vi "test_moteur.vi"() -> ()   [LabVIEW 2023]
panel:
  in  "WRITE PARAM":bool
  in  "param":T1
  out "param out":T1
  in  "READ PARAM":bool
  out "error out 2":errorcluster
  out "Serial Settings:Number of Bytes at Serial Port":u32
  in  "READ":bool
  out "read buffer":string
  in  "WRITE":bool
  in  "stop":bool
  in  "write buffer":string
  in  "VISA resource name":refnum<visa-resource-name>
  out "error out":errorcluster
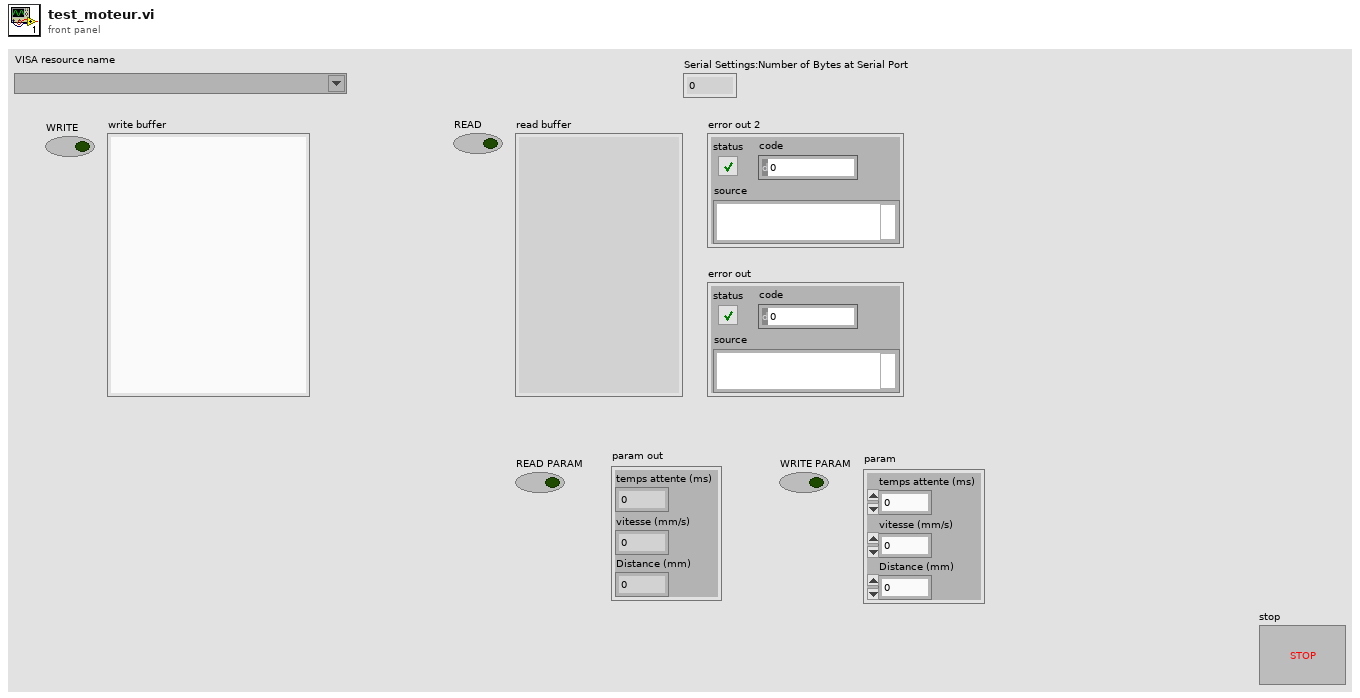
[diagram p1: front panel]
types:
  T1 = cluster{"temps attente (ms)":i32, "vitesse (mm/s)":dbl, "Distance (mm)":dbl}
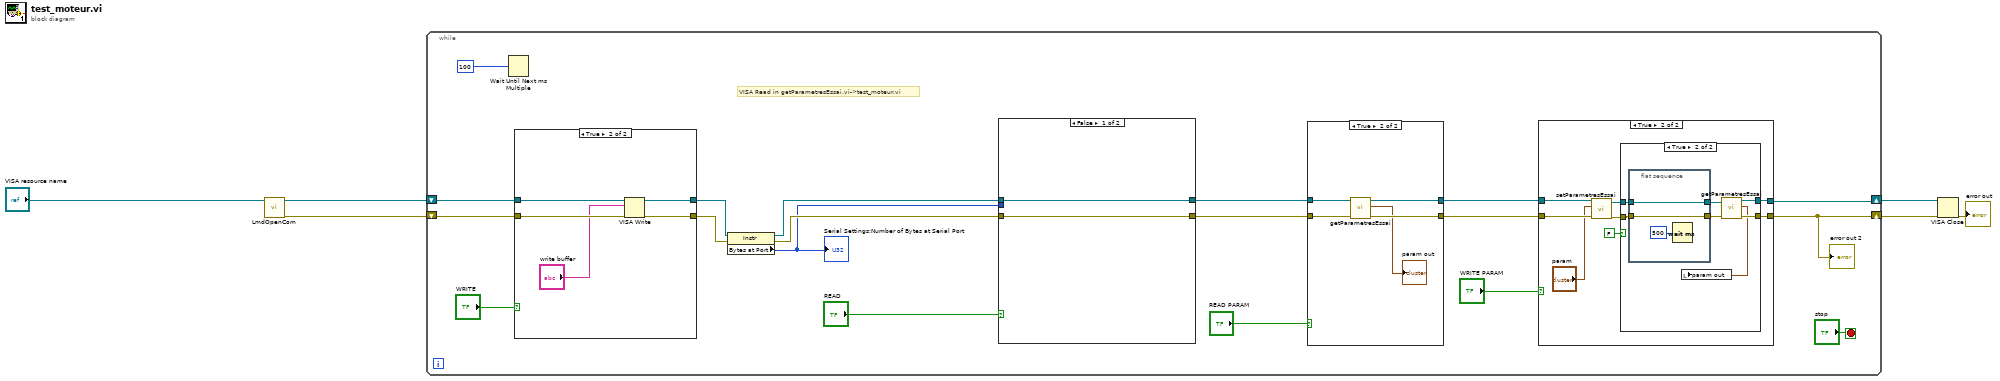
[diagram p0: block diagram]
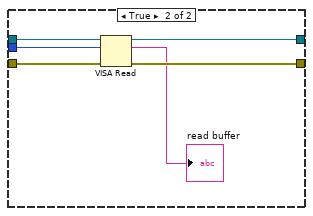
[diagram p5: hidden frame]
diagram:
  n1 = call "LmdOpenCom.vi"("VISA Refnum in"="VISA resource name") -> ("error out"=w5:errorcluster, "VISA Refnum out"=w1:refnum<visa-resource-name>)  [unwired: 9 in]
  n2 = while {
    shift-right: [w8] -> w3
    shift-left: w1 -> [w25]
    shift-right: [w9] -> w4
    shift-left: w5 -> [w24]
    stop <- "stop" stop-if-true
    # "VISA Read in getParametresEssai.vi->test_moteur.vi"
    n3 = Wait Until Next ms Multiple(millisecond multiple=u32 100) -> ()  [unwired: 1 out]
    n4 = case shown="True" "WRITE" {
      tunnel: w25 -> [w64 w69]
      tunnel: w24 -> [w63 w68]
      tunnel: [w63 w67] -> w19
      tunnel: [w64 w66] -> w20
      frame False {
      }
      frame True {
        n5 = VISA Write(VISA resource name=w69, write buffer="write buffer", error in (no error)=w68) -> (VISA resource name out=w66:refnum<visa-resource-name>, error out=w67:errorcluster)  [unwired: 1 out]
      }
    }
    n6 = property class="Instr"(reference=w20, error in=w19) -> (reference out=w17:refnum<visa-resource-name>, error out=w18:errorcluster, "Bytes at Port"=w15:u32)
    "Serial Settings:Number of Bytes at Serial Port" <- w15
    n7 = case shown="False" "READ" {
      tunnel: [w56 w60] -> w13
      tunnel: w18 -> [w56 w61]
      tunnel: [w55 w59] -> w12
      tunnel: w17 -> [w55 w62]
      tunnel: w15 -> [_ w57]
      frame False {
      }
      frame True {
        n8 = VISA Read(VISA resource name=w62, byte count=w57, error in (no error)=w61) -> (VISA resource name out=w59:refnum<visa-resource-name>, read buffer=→"read buffer":string, error out=w60:errorcluster)  [unwired: 1 out]
      }
    }
    n9 = case shown="True" "READ PARAM" {
      tunnel: w13 -> [w48 w54]
      tunnel: w12 -> [w49 w53]
      tunnel: [w49 w52] -> w10
      tunnel: [w48 w51] -> w11
      frame False {
      }
      frame True {
        n10 = call "getParametresEssai.vi"("error in (no error)"=w54, "VISA resource name"=w53) -> ("error out"=w51:errorcluster, "param out"=→"param out":T1, "VISA resource name out"=w52:refnum<visa-resource-name>)  [unwired: 7 in]
      }
    }
    n11 = case shown="True" "WRITE PARAM" {
      tunnel: w11 -> [w26 w35]
      tunnel: w10 -> [w27 w34]
      tunnel: [w26 w31] -> w9
      tunnel: [w27 w32] -> w8
      frame False {
      }
      frame True {
        n12 = call "setParametresEssai.vi"("error in (no error)"=w35, "param"="param", "VISA resource name"=w34) -> ("error out"=w29:errorcluster, "VISA resource name out"=w30:refnum<visa-resource-name>)  [unwired: 7 in]
        n13 = case shown="True" FALSE {
          tunnel: [w37 w44] -> w32
          tunnel: [w36 w43] -> w31
          tunnel: w30 -> [w37 w41]
          tunnel: w29 -> [w36 w38]
          frame False {
          }
          frame True {
            n14 = flat-sequence {
              tunnel: w41 -> [w47]
              tunnel: [w47] -> w40
              tunnel: [w46] -> w39
              tunnel: w38 -> [w46]
              frame #0 {
                n15 = Wait (ms)(milliseconds to wait=u32 500) -> ()  [unwired: 1 out]
              }
            }
            n16 = call "getParametresEssai.vi"("error in (no error)"=w39, "VISA resource name"=w40) -> ("error out"=w43:errorcluster, "param out"=w42:T1, "VISA resource name out"=w44:refnum<visa-resource-name>)  [unwired: 7 in]
            n17 = local write "param out"(w42) -> ()
          }
        }
      }
    }
    "error out 2" <- w9
  }
  n18 = VISA Close(VISA resource name=w3, error in (no error)=w4) -> (error out=→"error out":errorcluster)
